vi "Database Delete.vi"() -> ()   [LabVIEW 2012]
doc: "This example demonstrates how to use the DB Tools Delete Data VI to delete specific data from a database, located at LabVIEW\\examples\\database\\LabVIEW.mdb.\n\nThis example first creates a table, named DeleteData, in the database and inserts some randomly generated numbers to the table. This example then uses the DB Tools Delete Data VI to delete all numbers that equal the numeric value 1. The <B>Before</B> and <B>After</B> arrays display the original data and the remaining data, respectively."
uses:
  NI_Database_API_64.lvlib
  <vilib>/Utility/error.llb/DialogType.ctl
  _DB Variant To Data/Database Variant To Data.xnode
  Connection.llb/DB Tools Open Connec (Path).vi
panel:
  out "After":string[][](array[string])
  out "Before":string[][](array[string])
  # "Run this VI to see how this example deletes data from a database. The Before array displays the original data contained in the database. This example deletes all data that equals 1. The After array displays the remaining data contained in the database."
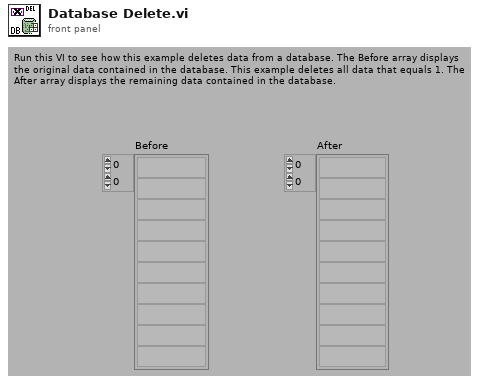
[diagram p1: front panel]
types:
  T1 = typedef "DialogType.ctl" = u16
  T2 = typedef "NI_Database_API_64.lvlib/Conn ObjectReference.ctl" = refnum<k1>
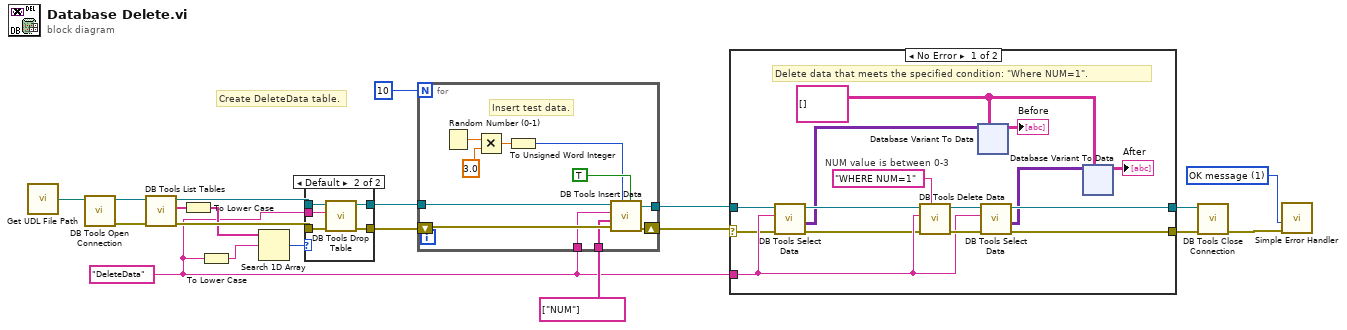
[diagram p0: block diagram]
diagram:
  w1 = "DeleteData" ("Table")
  w17 = T1 1 items=["no dialog", "OK message", "continue or stop message", "OK message + warnings", "continue/stop + warnings"] ("type of dialog (OK msg:1)")
  # "Create DeleteData table."
  n1 = call "Get UDL File Path.vi"() -> ("UDL file path"=w2:path)  [unwired: 1 in]
  n2 = call-poly "DB Tools Open Connection.vi"("connection information"=w2) -> ("error out"=w6:errorcluster, "connection reference"=w7:T2)  [unwired: 7 in]
  n3 = call "DB Tools List Tables.vi"("error in (no error)"=w6, "connection reference"=w7) -> ("error out"=w12:errorcluster, "tables"=w11:string[], "connection reference out"=w13:T2)  [unwired: 3 in]
  n4 = To Lower Case(string=w11) -> (all lower case string=w9:string[])
  n5 = To Lower Case(string=w1) -> (all lower case string=w10:string)
  n6 = Search 1D Array(1D array=w9, element=w10) -> (index of element=w8:i32)  [unwired: 1 in]
  n7 = case shown="Default" w8 {
    tunnel: w12 -> [w21 w27]
    tunnel: w13 -> [w22 w26]
    tunnel: [w22 w25] -> w5
    tunnel: [w21 w24] -> w4
    tunnel: w1 -> [_ w23]
    frame -1 {
    }
    frame Default {
      n8 = call "DB Tools Drop Table.vi"("error in (no error)"=w27, "table"=w23, "connection reference"=w26) -> ("error out"=w24:errorcluster, "connection reference out"=w25:T2)  [unwired: 5 in]
    }
  }
  n9 = for {
    N: 10 -> [_]
    tunnel: [w36] -> w15
    shift-right: [w37] -> w16
    shift-left: w4 -> [w38]
    tunnel: w5 -> [w31]
    tunnel: w1 -> [w30]
    tunnel: string[] ["NUM"] ("columns") -> [w29]
    # "Insert test data."
    n10 = Random Number (0-1)() -> (number: 0 to 1=w34:dbl)
    n11 = Multiply(x=w34, y=3.0) -> (x*y=w32:dbl)
    n12 = To Unsigned Word Integer(number=w32) -> (unsigned 16bit integer=w28:u16)
    n13 = call "DB Tools Insert Data.vi"("create table? (F)"=TRUE ("create table? (f)"), "data"=w28, "error in (no error)"=w38, "columns"=w29, "table"=w30, "connection reference"=w31) -> ("error out"=w37:errorcluster, "connection reference out"=w36:T2)  [unwired: 4 in]
  }
  n14 = case shown="No Error" w16 {
    selector: w16 -> [w40 w143]
    tunnel: [w53 w142] -> w20
    tunnel: [w52 w143] -> w19
    tunnel: w15 -> [w49 w142]
    tunnel: w1 -> [w44 _]
    frame No Error {
      w43 = string[][] []
      # "Delete data that meets the specified condition: \"Where NUM=1\"."
      # "NUM value is between 0-3"
      n15 = call "DB Tools Select Data.vi"("error in (no error)"=w40, "table"=w44, "connection reference"=w49) -> ("error out"=w39:errorcluster, "data"=w46:variant[][], "connection reference out"=w48:T2)  [unwired: 3 in]
      n16 = call "DB Tools Delete Data.vi"("condition"="WHERE NUM=1" ("delete optional clause"), "error in (no error)"=w39, "table"=w44, "connection reference"=w48) -> ("error out"=w50:errorcluster, "connection reference out"=w51:T2)  [unwired: 6 in]
      n17 = xnode "Database Variant To Data"("database variant"=w46, "type"=w43) -> ("data"=→"Before":string[][])  [unwired: 1 in, 1 out]
      n18 = call "DB Tools Select Data.vi"("error in (no error)"=w50, "table"=w44, "connection reference"=w51) -> ("error out"=w52:errorcluster, "data"=w45:variant[][], "connection reference out"=w53:T2)  [unwired: 3 in]
      n19 = xnode "Database Variant To Data"("database variant"=w45, "type"=w43) -> ("data"=→"After":string[][])  [unwired: 1 in, 1 out]
    }
    frame Error {
    }
  }
  n20 = call "DB Tools Close Connection.vi"("error in (no error)"=w19, "connection reference"=w20) -> ("error out"=w18:errorcluster)  [unwired: 5 in]
  n21 = call <vilib>:"Simple Error Handler.vi"("type of dialog (OK msg:1)"=w17, "error in (no error)"=w18) -> ()  [unwired: 3 in, 5 out]
